vi "Finish.vi"   [LabVIEW 2015]
doc: "This VI is called just before exiting. It is expected to close I/O refnum, save collected data, etc."
uses:
  Device Refnums.ctl
  <vilib>/Rock Robotics/WPI/Utilities/WPI_GetSetVariantRefNum.vi
  <vilib>/Rock Robotics/WPI/Ultrasonic/WPI_SonarMB1010DigitalRefNum Registry Get.vi
  <vilib>/Rock Robotics/WPI/Ultrasonic/WPI_SonarMB1010DigitalClose.vi
  ADIS16448-RoboRIO-Driver.git/trunk/LabVIEW/ADI MXP IMU/FRC_ADIS16448_IMU.lvlib
types:
  T1 = typedef "Device Refnums.ctl" = string
  T2 = typedef "WPI_MotorControlDeviceRef.ctl" = cluster{"DeviceStatus":errorcluster, "Type":T3, "PWM":cluster{"PWM Channel":T4, "DeadBand":T5}, "CAN":cluster{"Device Number":u8, "Control Mode":T6, "Semaphore":T7, "Max Vout":dbl, "TalonSRX Control Mode":T8}, "Invert":bool}
  T3 = typedef "WPI_MotorControlType.ctl" = enum16{"PWM", "CAN", "CANTalonSRX"}
  T4 = typedef "FPGA_DIOPWMChannel.ctl" = enum8{"PWM 0", "PWM 1", "PWM 2", "PWM 3", "PWM 4", "PWM 5", "PWM 6", "PWM 7", "PWM 8", "PWM 9", "PWM MXP 0", "PWM MXP 1", "PWM MXP 2", "PWM MXP 3", "PWM MXP 4", "PWM MXP 5", "PWM MXP 6", "PWM MXP 7", "PWM MXP 8", "PWM MXP 9", "Invalid"}
  T5 = typedef "WPI_PWMDeadband.ctl" = cluster{"Name":string, "maxPositivePwm":i32, "minPositivePwm":i32, "centerPwm":i32, "maxNegativePwm":i32, "minNegativePwm":i32, "angularRange":u16}
  T6 = typedef "WPI_CANJaguar_ControlMode.ctl" = enum8{"Percent VBus", "Current", "Speed", "Position", "Voltage"}
  T7 = typedef "Semaphore RefNum" = refnum<k1>
  T8 = typedef "WPI_CANTalonSRX_APIControlMode.ctl" = enum8{"Percent VBus", "Speed", "Position", "Slave", "Unchanged / Invalid", "Voltage Compensation", "Current", "Motion Profile"}
  T9 = typedef "WPI_JoystickDevRef.ctl" = cluster{"Device":T10}
  T10 = typedef "WPI_JoystickDeviceEnum.ctl" = enum16{"USB 0", "USB 1", "USB 2", "USB 3", "USB 4", "USB 5"}
  T11 = typedef "WPI_RobotDriveDevRef.ctl" = cluster{"DevStatus":errorcluster, "Motors[]":T2[], "Square Inputs":bool, "Max Output":dbl}
  T12 = typedef "WPI_EncoderDevRef.ctl" = cluster{"DevStatus":errorcluster, "EncoderIndex":T13, "CounterIndex":T14, "DistancePerCount":dbl, "Decoding Type":T15}
  T13 = typedef "FPGA_EncoderIdx.ctl" = enum8{"Enc 0", "Enc 1", "Enc 2", "Enc 3", "Enc 4", "Enc 5", "Enc 6", "Enc 7", "Invalid"}
  T14 = typedef "FPGA_CounterCtrSystemIndex.ctl" = enum8{"Ctr 0", "Ctr 1", "Ctr 2", "Ctr 3", "Ctr 4", "Ctr 5", "Ctr 6", "Ctr 7", "Invalid"}
  T15 = typedef "WPI_EncoderType.ctl" = enum16{"1x", "2x", "4x"}
  T16 = typedef "WPI_SwitchDevRef.ctl" = cluster{"DevStatus":errorcluster, "DIO Channel":T17, "CntIndex":T14, "Normally Closed":bool}
  T17 = typedef "FPGA_DIOChannel.ctl" = enum8{"DIO 0", "DIO 1", "DIO 2", "DIO 3", "DIO 4", "DIO 5", "DIO 6", "DIO 7", "DIO 8", "DIO 9", "DIO MXP 0", "DIO MXP 1", "DIO MXP 2", "DIO MXP 3", "DIO MXP 4", "DIO MXP 5", "DIO MXP 6", "DIO MXP 7", "DIO MXP 8", "DIO MXP 9", "DIO MXP 10", "DIO MXP 11", "DIO MXP 12", "DIO MXP 13", "DIO MXP 14", "DIO MXP 15", "Invalid"}
  T18 = typedef "WPI_SonarMB1010DigitalDeviceRef.ctl" = cluster{"CounterDevRef":T19, "Scaling factor (s/in)":dbl}
  T19 = typedef "WPI_CounterDevRef.ctl" = cluster{"DevStatus":errorcluster, "CntIndex":T14}
  T20 = typedef "WPI_AnalogChannelDevRef.ctl" = cluster{"DevStatus":errorcluster, "Analog Channel":T21}
  T21 = typedef "FPGA_AIChannel.ctl" = enum8{"AI 0", "AI 1", "AI 2", "AI 3", "AI MXP 0", "AI MXP 1", "AI MXP 2", "AI MXP 3", "Invalid"}
  T22 = typedef "WPI_SolenoidDevRef.ctl" = cluster{"DevStatus":errorcluster, "Pneumatics Control Module":u8, "Forward Solenoid Channel":T23, "Reverse Solenoid Channel":T23}
  T23 = typedef "WPI_SolenoidChannel.ctl" = enum8{"Solenoid 0", "Solenoid 1", "Solenoid 2", "Solenoid 3", "Solenoid 4", "Solenoid 5", "Solenoid 6", "Solenoid 7", "Invalid"}
  T24 = typedef "WPI_CompressorDevRef.ctl" = cluster{"DevStatus":errorcluster, "Pneumatics Control Module":u8}
  T25 = typedef "FRC_ADIS16448_IMU.lvlib/WPI_IMU_ADIS16448_InterruptDevRef.ctl" = cluster{"ADI IMU DevRef":T26, "InterruptRef":T28}
  T26 = typedef "FRC_ADIS16448_IMU.lvlib/WPI_IMU_ADIS16448_IMUDevRef.ctl" = cluster{"DevStatus":errorcluster, "Handle":i32, "SPI Bus":T27, "Device Found":bool, "Device Ready":bool, "Yaw Axis":enum16{"X", "Y", "Z"}, "AHRS Algorithm":enum16{"Complementary", "Madgwick"}, "Serial":u16, "Lot ID 2":u16, "Lot ID 1":u16, "Product ID":u16}
  T27 = typedef "spi_bus.ctl" = enum16{"SPI On-Board, CS0", "SPI On-Board, CS1", "SPI On-Board, CS2", "SPI On-Board, CS3", "SPI MXP", "Invalid"}
  T28 = typedef "WPI_InterruptRef.ctl" = cluster{"DevStatus":errorcluster, "InterruptIndex":T29}
  T29 = typedef "FPGA_InterruptIndex.ctl" = enum8{"0", "1", "2", "3", "4", "5", "6", "7", "Invalid"}
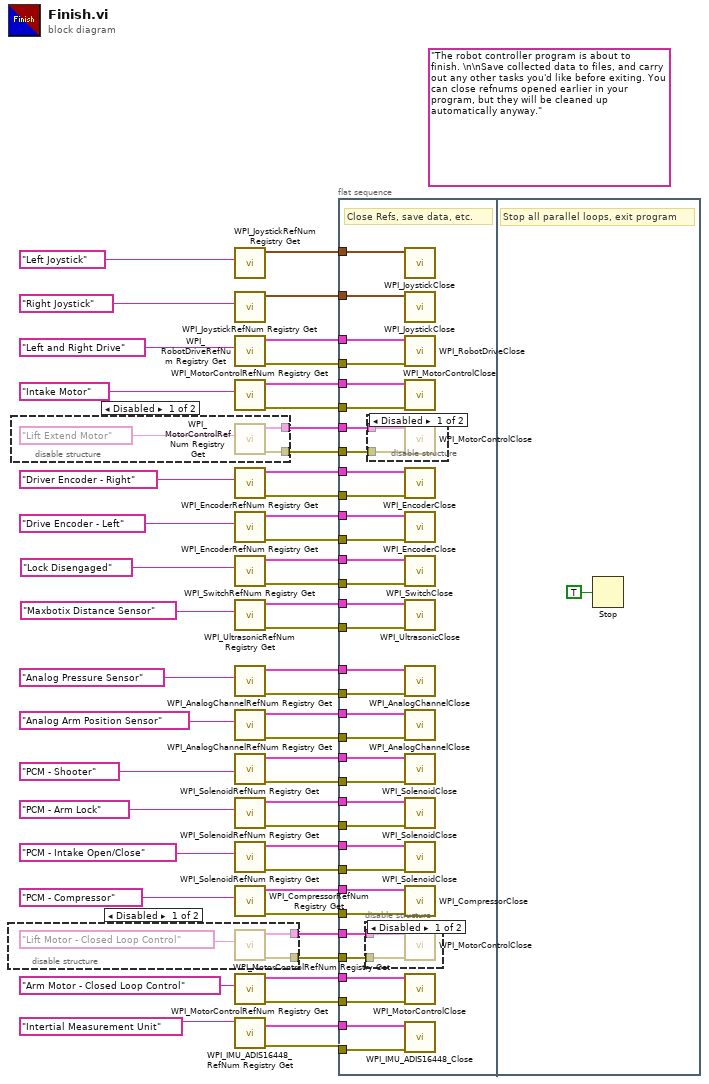
[diagram p0: block diagram]
diagram:
  (unwired) "The robot controller program is about to finish. \n\nSave collected data to files, and carry out any other tasks you'd like before exiting. You can close refnums opened earlier in your program, but they will be cleaned up automatically anyway."
  n1 = disable-structure shown="Disabled" {
    disable-tunnel: [w53 _] -> w46
    disable-tunnel: [w51 _] -> w20
    frame Disabled {
      n2 = call <vilib>:"WPI_MotorControlRefNum Registry Get.vi"("refnum name"=T1 "Lift Motor - Closed Loop Control" ("Device Name")) -> ("error out"=w51:errorcluster, "MotorControlDevRef"=w53:T2)  [unwired: 9 in]
    }
    frame Enabled {
    }
  }
  n3 = disable-structure shown="Disabled" {
    disable-tunnel: [w56 _] -> w43
    disable-tunnel: [w54 _] -> w24
    frame Disabled {
      n4 = call <vilib>:"WPI_MotorControlRefNum Registry Get.vi"("refnum name"=T1 "Lift Extend Motor" ("Device Name")) -> ("error out"=w54:errorcluster, "MotorControlDevRef"=w56:T2)  [unwired: 9 in]
    }
    frame Enabled {
    }
  }
  n5 = call <vilib>:"WPI_JoystickRefNum Registry Get.vi"("refnum name"=T1 "Left Joystick" ("Device Name")) -> ("JoystickDevRef"=w29:T9)  [unwired: 9 in, 1 out]
  n6 = call <vilib>:"WPI_JoystickRefNum Registry Get.vi"("refnum name"=T1 "Right Joystick" ("Device Name")) -> ("JoystickDevRef"=w30:T9)  [unwired: 9 in, 1 out]
  n7 = call <vilib>:"WPI_RobotDriveRefNum Registry Get.vi"("refnum name"=T1 "Left and Right Drive" ("Device Name")) -> ("error out"=w25:errorcluster, "RobotDriveDevRef"=w50:T11)  [unwired: 1 in, 8 out]
  n8 = call <vilib>:"WPI_MotorControlRefNum Registry Get.vi"("refnum name"=T1 "Intake Motor" ("Device Name")) -> ("error out"=w26:errorcluster, "MotorControlDevRef"=w42:T2)  [unwired: 9 in]
  n9 = call <vilib>:"WPI_EncoderRefNum Registry Get.vi"("refnum name"=T1 "Driver Encoder - Right" ("Device Name")) -> ("error out"=w23:errorcluster, "EncoderDevRef"=w44:T12)  [unwired: 9 in]
  n10 = call <vilib>:"WPI_EncoderRefNum Registry Get.vi"("refnum name"=T1 "Drive Encoder - Left" ("Device Name")) -> ("error out"=w22:errorcluster, "EncoderDevRef"=w45:T12)  [unwired: 9 in]
  n11 = call <vilib>:"WPI_SwitchRefNum Registry Get.vi"("refnum name"=T1 "Lock Disengaged" ("Device Name")) -> ("error out"=w13:errorcluster, "SwitchDevRef"=w11:T16)  [unwired: 9 in]
  n12 = call-poly <vilib>:"WPI_UltrasonicRefNum Registry Get.vi"("refnum name"=T1 "Maxbotix Distance Sensor" ("Device Name")) -> ("error out"=w8:errorcluster, "SonarMB1010DigitalDevRef"=w9:T18)  [unwired: 9 in]
  n13 = call <vilib>:"WPI_AnalogChannelRefNum Registry Get.vi"("refnum name"=T1 "Analog Pressure Sensor" ("Device Name")) -> ("error out"=w17:errorcluster, "AIDeviceRef"=w1:T20)  [unwired: 9 in]
  n14 = call <vilib>:"WPI_AnalogChannelRefNum Registry Get.vi"("refnum name"=T1 "Analog Arm Position Sensor" ("Device Name")) -> ("error out"=w7:errorcluster, "AIDeviceRef"=w6:T20)  [unwired: 9 in]
  n15 = call <vilib>:"WPI_SolenoidRefNum Registry Get.vi"("refnum name"=T1 "PCM - Shooter" ("Device Name")) -> ("error out"=w19:errorcluster, "SolenoidDevRef"=w48:T22)  [unwired: 9 in]
  n16 = call <vilib>:"WPI_SolenoidRefNum Registry Get.vi"("refnum name"=T1 "PCM - Arm Lock" ("Device Name")) -> ("error out"=w21:errorcluster, "SolenoidDevRef"=w47:T22)  [unwired: 9 in]
  n17 = call <vilib>:"WPI_SolenoidRefNum Registry Get.vi"("refnum name"=T1 "PCM - Intake Open/Close" ("Device Name")) -> ("error out"=w4:errorcluster, "SolenoidDevRef"=w3:T22)  [unwired: 9 in]
  n18 = call <vilib>:"WPI_CompressorRefNum Registry Get.vi"("refnum name"=T1 "PCM - Compressor" ("Device Name")) -> ("error out"=w18:errorcluster, "CompressorDevRef"=w49:T24)  [unwired: 9 in]
  n19 = call <vilib>:"WPI_MotorControlRefNum Registry Get.vi"("refnum name"=T1 "Arm Motor - Closed Loop Control" ("Device Name")) -> ("error out"=w16:errorcluster, "MotorControlDevRef"=w15:T2)  [unwired: 9 in]
  n20 = call "WPI_IMU_ADIS16448_RefNum Registry Get.vi"("refnum name"=T1 "Intertial Measurement Unit" ("Device Name")) -> ("error out"=w41:errorcluster, "ADI IMU Interrupt DevRef"=w40:T25)  [unwired: 9 in]
  n21 = flat-sequence {
    tunnel: w50 -> [w90]
    tunnel: w42 -> [w89]
    tunnel: w43 -> [w88]
    tunnel: w1 -> [w87]
    tunnel: w49 -> [w86]
    tunnel: w48 -> [w85]
    tunnel: w47 -> [w84]
    tunnel: w46 -> [w83]
    tunnel: w45 -> [w82]
    tunnel: w44 -> [w81]
    tunnel: w41 -> [w80]
    tunnel: w40 -> [w79]
    tunnel: w30 -> [w78]
    tunnel: w29 -> [w77]
    tunnel: w26 -> [w76]
    tunnel: w25 -> [w75]
    tunnel: w24 -> [w74]
    tunnel: w23 -> [w73]
    tunnel: w22 -> [w72]
    tunnel: w21 -> [w71]
    tunnel: w20 -> [w70]
    tunnel: w19 -> [w69]
    tunnel: w18 -> [w68]
    tunnel: w17 -> [w67]
    tunnel: w16 -> [w66]
    tunnel: w15 -> [w65]
    tunnel: w13 -> [w64]
    tunnel: w11 -> [w63]
    tunnel: w9 -> [w62]
    tunnel: w8 -> [w61]
    tunnel: w6 -> [w59]
    tunnel: w7 -> [w60]
    tunnel: w3 -> [w57]
    tunnel: w4 -> [w58]
    frame #0 {
      # "Close Refs, save data, etc."
      n22 = disable-structure shown="Disabled" {
        disable-tunnel: w83 -> [w94 _]
        disable-tunnel: w70 -> [w93 _]
        frame Disabled {
          n23 = call <vilib>:"WPI_MotorControlClose.vi"("error in (no error)"=w93, "MotorControlDevRef"=w94) -> ()  [unwired: 9 in, 1 out]
        }
        frame Enabled {
        }
      }
      n24 = disable-structure shown="Disabled" {
        disable-tunnel: w88 -> [w92 _]
        disable-tunnel: w74 -> [w91 _]
        frame Disabled {
          n25 = call <vilib>:"WPI_MotorControlClose.vi"("error in (no error)"=w91, "MotorControlDevRef"=w92) -> ()  [unwired: 9 in, 1 out]
        }
        frame Enabled {
        }
      }
      n26 = call <vilib>:"WPI_JoystickClose.vi"("JoystickDevRef"=w77) -> ()  [unwired: 11 in]
      n27 = call <vilib>:"WPI_JoystickClose.vi"("JoystickDevRef"=w78) -> ()  [unwired: 11 in]
      n28 = call <vilib>:"WPI_RobotDriveClose.vi"("error in (no error)"=w75, "RobotDriveDevRef"=w90) -> ()  [unwired: 10 out]
      n29 = call <vilib>:"WPI_MotorControlClose.vi"("error in (no error)"=w76, "MotorControlDevRef"=w89) -> ()  [unwired: 9 in, 1 out]
      n30 = call <vilib>:"WPI_EncoderClose.vi"("error in (no error)"=w73, "EncoderDevRef"=w81) -> ()  [unwired: 9 in, 1 out]
      n31 = call <vilib>:"WPI_EncoderClose.vi"("error in (no error)"=w72, "EncoderDevRef"=w82) -> ()  [unwired: 9 in, 1 out]
      n32 = call <vilib>:"WPI_SwitchClose.vi"("error in (no error)"=w64, "SwitchDevRef"=w63) -> ()  [unwired: 9 in, 1 out]
      n33 = call-poly <vilib>:"WPI_UltrasonicClose.vi"("error in (no error)"=w61, "SonarMB1010DigitalDevRef"=w62) -> ()  [unwired: 9 in, 1 out]
      n34 = call <vilib>:"WPI_AnalogChannelClose.vi"("error in (no error)"=w67, "AIDeviceRef"=w87) -> ()  [unwired: 9 in, 1 out]
      n35 = call <vilib>:"WPI_AnalogChannelClose.vi"("error in (no error)"=w60, "AIDeviceRef"=w59) -> ()  [unwired: 9 in, 1 out]
      n36 = call <vilib>:"WPI_SolenoidClose.vi"("error in (no error)"=w69, "SolenoidDevRef"=w85) -> ()  [unwired: 9 in, 1 out]
      n37 = call <vilib>:"WPI_SolenoidClose.vi"("error in (no error)"=w71, "SolenoidDevRef"=w84) -> ()  [unwired: 9 in, 1 out]
      n38 = call <vilib>:"WPI_SolenoidClose.vi"("error in (no error)"=w58, "SolenoidDevRef"=w57) -> ()  [unwired: 9 in, 1 out]
      n39 = call <vilib>:"WPI_CompressorClose.vi"("error in (no error)"=w68, "CompressorDevRef"=w86) -> ()  [unwired: 9 in, 1 out]
      n40 = call <vilib>:"WPI_MotorControlClose.vi"("error in (no error)"=w66, "MotorControlDevRef"=w65) -> ()  [unwired: 9 in, 1 out]
      n41 = call "WPI_IMU_ADIS16448_Close.vi"("error in"=w80, "ADI IMU Interrupt DevRef"=w79) -> ()  [unwired: 9 in, 1 out]
    }
    frame #1 {
      # "Stop all parallel loops, exit program"
      n42 = Stop(stop? (T)=TRUE ("Quit")) -> ()
    }
  }
